vi "UE9 Stream with Stream-DAC with mid-stream update.vi"() -> ()   [LabVIEW 2021]
panel:
  in  "DAC1 # Update Points (0-128":i32=2
  in  "DAC0 # Update Points (0-128)":i32=10
  in  "DAC Data":dbl[][](array[numeric])=[[0.0, 0.0], [1.0, 5.0], [2.0, 0.0], [3.0, 0.0], [4.0, 0.0], [5.0, 0.0], [4.0, 0.0], [3.0, 0.0], [2.0, 0.0], [1.0, 0.0]] format="%.3f"
  out "Actual Scan Rate (Hz)":dbl=1000.0 format="%.3f"
  out "# Scans Read":i32
  out "# of iterations":i32
  out "AIN0 Data":dbl[](array[numeric]) format="%.3f"
  in  "Scan Rate (Hz)":dbl=1000.0 format="%.3f"
  in  "stop":bool
  out "Error Message":string
  # "This example streams from AIN0 using the\nfirst found USB UE9.  Updates both DACs\nat the same rate.\n\nRequires Control firmware V1.94 or higher."
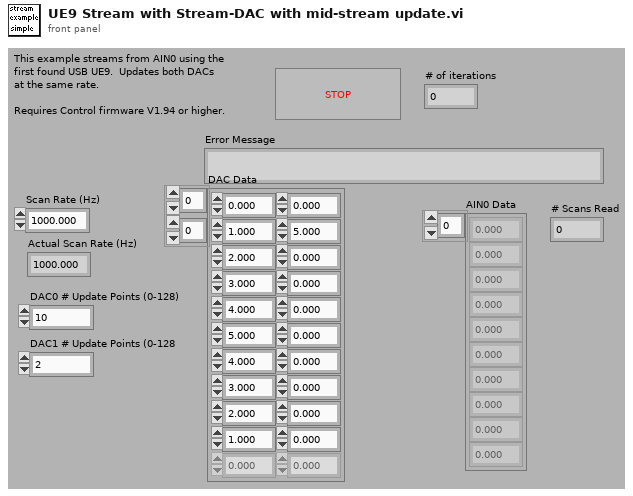
[diagram p1: front panel]
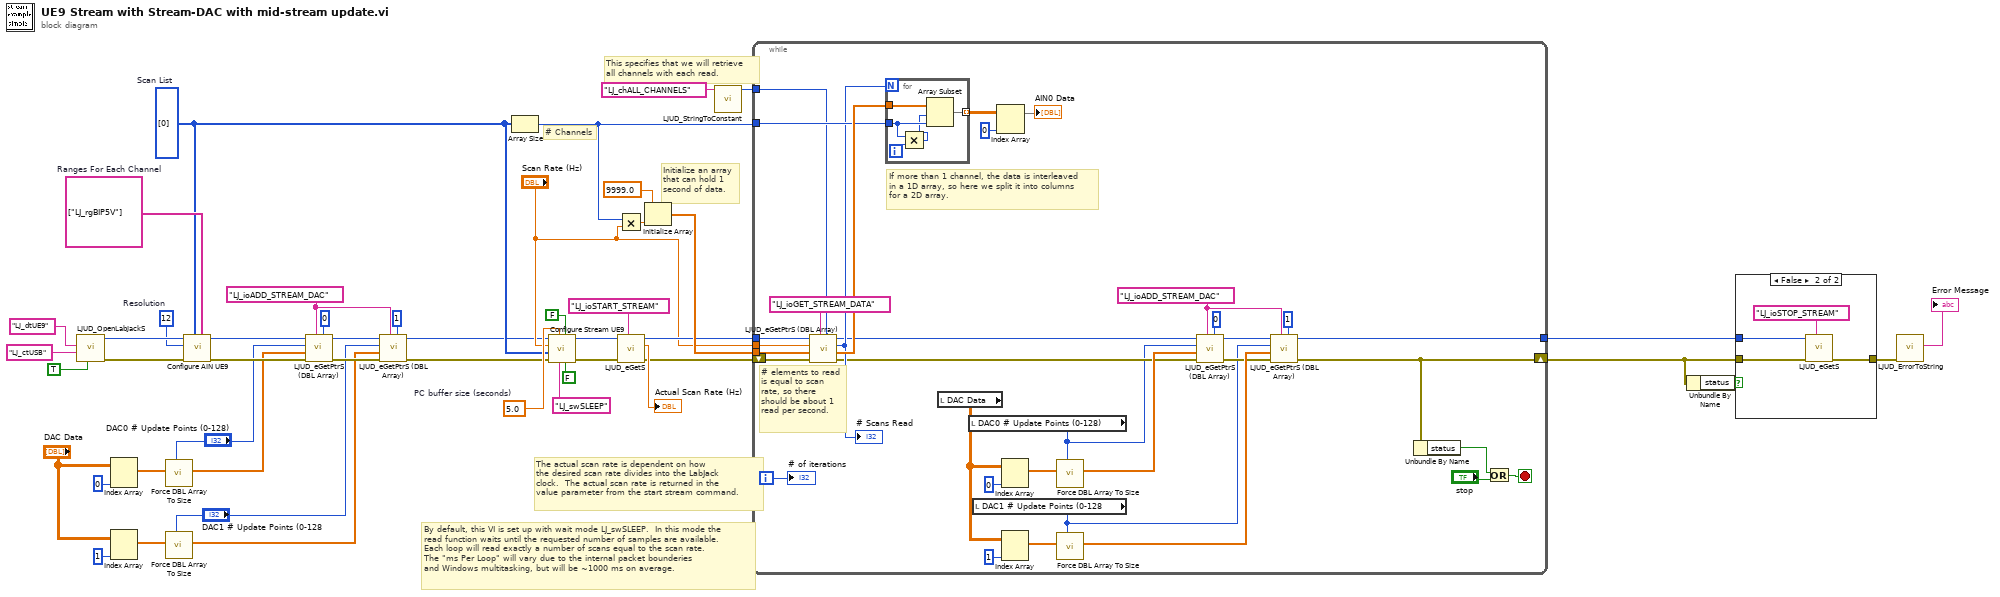
[diagram p0: block diagram]
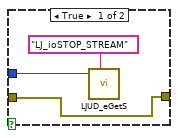
[diagram p2: hidden frame]
diagram:
  w1 = "LJ_ioADD_STREAM_DAC" ("IOType")
  w24 = 12  # Resolution
  w25 = i32[] [0]  # Scan List
  w26 = string[] ["LJ_rgBIP5V"]  # Ranges For Each Channel
  w37 = 5.0  # PC buffer size (seconds)
  # "Initialize an array\nthat can hold 1\nsecond of data."
  # "# Channels"
  # "This specifies that we will retrieve\nall channels with each read."
  # "The actual scan rate is dependent on how\nthe desired scan rate divides into the LabJack\nclock.  The actual scan rate is returned in the\nvalue parameter from the start stream command."
  # "By default, this VI is set up with wait mode LJ_swSLEEP.  In this mode the\nread function waits until the requested number of samples are available.\nEach loop will read exactly a number of scans equal to the scan rate.\nThe \"ms Per Loop\" will vary due to the internal packet bounderies\nand Windows multitasking, but will be ~1000 ms on average."
  n1 = call "LJUD_OpenLabJackS.vi"("FirstFound"=TRUE, "ConnectionType"="LJ_ctUSB", "DeviceType"="LJ_dtUE9") -> ("error out"=w33:errorcluster, "Handle"=w32:i32)  [unwired: 6 in, 1 out]
  n2 = Index Array(array="DAC Data", index (col)=0 ("Disabled Index (col)")) -> (element=w18:dbl[])  [unwired: 1 in]
  n3 = Index Array(array="DAC Data", index (col)=1 ("Disabled Index (col)")) -> (element=w17:dbl[])  [unwired: 1 in]
  n4 = call "Force DBL Array To Size.vi"("# Elements"="DAC0 # Update Points (0-128)", "DBL Array In"=w18) -> ("DBL Array Out"=w9:dbl[])  [unwired: 9 in]
  n5 = call "Force DBL Array To Size.vi"("# Elements"="DAC1 # Update Points (0-128", "DBL Array In"=w17) -> ("DBL Array Out"=w8:dbl[])  [unwired: 9 in]
  n6 = call "Configure AIN UE9.vi"("Ranges"=w26, "Channels"=w25, "error in"=w33, "Resolution"=w24, "Handle In"=w32) -> ("error out"=w13:errorcluster, "Handle Out"=w12:i32)  [unwired: 5 in]
  n7 = call "LJUD_eGetPtrS (DBL Array).vi"("Channel"=0, "IOType"=w1, "error in"=w13, "DBL Array Write"=w9, "Value"="DAC0 # Update Points (0-128)", "Handle In"=w12) -> ("error out"=w10:errorcluster, "Handle Out"=w11:i32)  [unwired: 2 in, 2 out]
  n8 = call "LJUD_eGetPtrS (DBL Array).vi"("Channel"=1, "IOType"=w1, "error in"=w10, "DBL Array Write"=w8, "Value"="DAC1 # Update Points (0-128", "Handle In"=w11) -> ("error out"=w2:errorcluster, "Handle Out"=w3:i32)  [unwired: 2 in, 2 out]
  n9 = Array Size(array=w25) -> (size(s)=w42:i32)
  n10 = call "Configure Stream UE9.vi"("External Scan Trigger"=FALSE, "Scan Clock Output"=FALSE, "Wait Mode"="LJ_swSLEEP" ("Wait Mode (2)"), "PC buffer size (seconds)"=w37, "error in"=w2, "Scan List"=w25, "Scan Rate (Hz)"="Scan Rate (Hz)", "Handle In"=w3) -> ("error out"=w46:errorcluster, "Handle Out"=w47:i32)  [unwired: 1 in, 1 out]
  n11 = Multiply(x=w42, y="Scan Rate (Hz)") -> (x*y=w45:dbl)
  n12 = call "LJUD_eGetS.vi"("IOType"="LJ_ioSTART_STREAM", "error in"=w46, "Handle In"=w47) -> ("error out"=w19:errorcluster, "Value Read"=→"Actual Scan Rate (Hz)":dbl, "Handle Out"=w31:i32)  [unwired: 6 in]
  n13 = Initialize Array(9999.0, w45) -> (w43:dbl[])
  n14 = call "LJUD_StringToConstant.vi"("String"="LJ_chALL_CHANNELS") -> ("Constant Number"=w27:i32)  [unwired: 9 in, 1 out]
  n15 = while {
    shift-left: w19 -> [w70]
    shift-right: [w55] -> w20
    tunnel: w27 -> [w73]
    tunnel: [w54] -> w40
    tunnel: w42 -> [w75]
    tunnel: w43 -> [w78]
    tunnel: "Scan Rate (Hz)" -> [w76]
    tunnel: w31 -> [w80]
    i -> [w74]
    stop <- w72 stop-if-true
    w66 = "LJ_ioADD_STREAM_DAC" ("IOType")
    # "If more than 1 channel, the data is interleaved\nin a 1D array, so here we split it into columns\nfor a 2D array."
    # "# elements to read\nis equal to scan\nrate, so there\nshould be about 1\nread per second."
    n16 = call "LJUD_eGetPtrS (DBL Array).vi"("Channel"=w73, "IOType"="LJ_ioGET_STREAM_DATA", "error in"=w70, "DBL Array Write"=w78, "Value"=w76, "Handle In"=w80) -> ("error out"=w52:errorcluster, "DBL Array Read"=w77:dbl[], "Value"=w71:i32, "Handle Out"=w53:i32)  [unwired: 2 in]
    "# Scans Read" <- w71
    n17 = for {
      N: w71 -> [_]
      tunnel: w77 -> [w87]
      tunnel: w75 -> [w86]
      tunnel: [w83] -> w69 mode=indexing
      i -> [w85]
      n18 = Multiply(x=w86, y=w85) -> (x*y=w84:i32)
      n19 = Array Subset(array=w87, index=w84, length=w86) -> (w83:dbl[])
    }
    n20 = local read "DAC Data"() -> (w51:dbl[][])
    n21 = local read "DAC0 # Update Points (0-128)"() -> (w50:i32)
    n22 = local read "DAC1 # Update Points (0-128"() -> (w49:i32)
    n23 = Index Array(array=w69, index (col)=0 ("Disabled Index (col)")) -> (element=→"AIN0 Data":dbl[])  [unwired: 1 in]
    n24 = Index Array(array=w51, index (col)=0 ("Disabled Index (col)")) -> (element=w56:dbl[])  [unwired: 1 in]
    n25 = Index Array(array=w51, index (col)=1 ("Disabled Index (col)")) -> (element=w57:dbl[])  [unwired: 1 in]
    n26 = call "Force DBL Array To Size.vi"("# Elements"=w50, "DBL Array In"=w56) -> ("DBL Array Out"=w62:dbl[])  [unwired: 9 in]
    n27 = call "Force DBL Array To Size.vi"("# Elements"=w49, "DBL Array In"=w57) -> ("DBL Array Out"=w63:dbl[])  [unwired: 9 in]
    n28 = call "LJUD_eGetPtrS (DBL Array).vi"("Channel"=0, "IOType"=w66, "error in"=w52, "DBL Array Write"=w62, "Value"=w50, "Handle In"=w53) -> ("error out"=w61:errorcluster, "Handle Out"=w60:i32)  [unwired: 2 in, 2 out]
    n29 = call "LJUD_eGetPtrS (DBL Array).vi"("Channel"=1, "IOType"=w66, "error in"=w61, "DBL Array Write"=w63, "Value"=w49, "Handle In"=w60) -> ("error out"=w55:errorcluster, "Handle Out"=w54:i32)  [unwired: 2 in, 2 out]
    n30 = Unbundle By Name(w55) -> ("status"=w81:bool)
    n31 = Or(x=w81, y="stop") -> (x .or. y?=w72:bool)
    "# of iterations" <- w74
  }
  n32 = Unbundle By Name(w20) -> ("status"=w29:bool)
  n33 = case shown="False" w29 {
    tunnel: w40 -> [w89 w93]
    tunnel: [w88 w92] -> w39
    tunnel: w20 -> [w88 w91]
    frame True {
      n34 = call "LJUD_eGetS.vi"("IOType"="LJ_ioSTOP_STREAM", "Handle In"=w89) -> ()  [unwired: 7 in, 3 out]
    }
    frame False {
      n35 = call "LJUD_eGetS.vi"("IOType"="LJ_ioSTOP_STREAM", "error in"=w91, "Handle In"=w93) -> ("error out"=w92:errorcluster)  [unwired: 6 in, 2 out]
    }
  }
  n36 = call "LJUD_ErrorToString.vi"("error in"=w39) -> ("String"=→"Error Message":string)  [unwired: 10 in]
